vi "Assert_Buffer_Is_File.vi"(10 "body":string) -> (2 "File":path, 3 "is File?":bool)   [LabVIEW 2020, in "REST Client.lvlib" / "REST Client.lvclass"]
uses:
  REST Client.lvclass
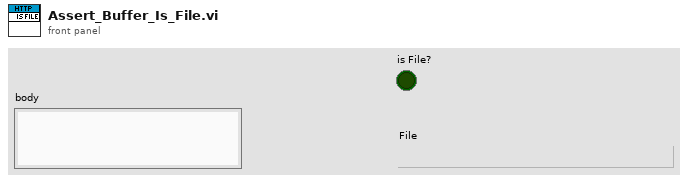
[diagram p1: front panel]
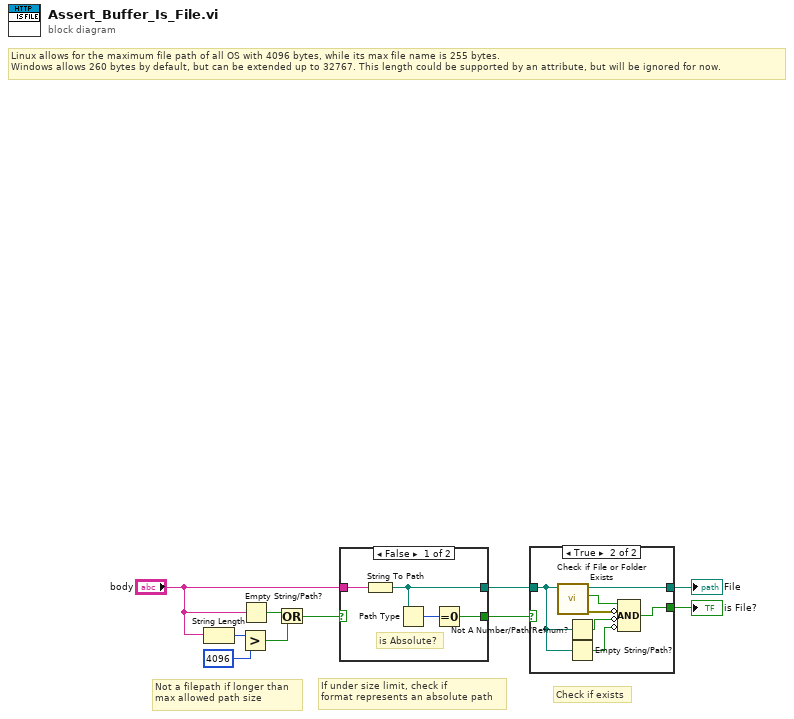
[diagram p0: block diagram]
diagram:
  # "Check if exists"
  # "If under size limit, check if\nformat represents an absolute path"
  # "Not a filepath if longer than\nmax allowed path size"
  # "Linux allows for the maximum file path of all OS with 4096 bytes, while its max file name is 255 bytes.\nWindows allows 260 bytes by default, but can be extended up to 32767. This length could be supported by an attribute, but will be ignored for now."
  n1 = String Length(string="body") -> (length=w8:i32)
  n2 = Greater?(x=w8, y=4096) -> (0:w7:bool)
  n3 = Empty String/Path?(string/path="body") -> (empty?=w6:bool)
  n4 = Or(x=w6, y=w7) -> (x .or. y?=w5:bool)
  n5 = case shown="False" w5 {
    tunnel: [w11 _] -> w3
    tunnel: "body" -> [w14 _]
    tunnel: [w12 _] -> w2
    frame False {
      # "is Absolute?"
      n6 = String To Path(string=w14) -> (path=w11:path)
      n7 = Path Type(1:w11) -> (0:w13:i16)
      n8 = Equal To 0?(x=w13) -> (x = 0?=w12:bool)
    }
    frame True {
    }
  }
  n9 = case shown="True" w2 {
    tunnel: w3 -> [_ w17]
    tunnel: [_ w19] -> w10
    tunnel: [_ w18] -> w9
    frame False {
      # "Not a filepath"
    }
    frame True {
      n10 = call <vilib>:"Check if File or Folder Exists.vi"("path"=w17) -> ("error out"=w20:errorcluster, "file or folder exists?"=w21:bool, "dup path"=w19:path)  [unwired: 8 in]
      n11 = Not A Number/Path/Refnum?(number/path/refnum=w17) -> (NaN/Path/Refnum?=w16:bool)
      n12 = Empty String/Path?(string/path=w17) -> (empty?=w15:bool)
      n13 = Compound Arithmetic op=AND(w21, invert w20, invert w16, invert w15) -> (w18:bool)
    }
  }
  "File" <- w10
  "is File?" <- w9
